vi "Open Handler.vi"(8 "error in (no error)":errorcluster, 10 "Configure Server":T1={"Outgoing Mail Server (SMTP)"="smtp.gmail.com", "Port"="587", "Sender's Email Address"="ltt24012025@gmail.com", "username"="ltt24012025@gmail.com", "password"="nftv\\swtbe\\suutg\\scqps", "Enable TLS"=TRUE}, 11 "Mail in":refnum<class "Mail.lvclass">) -> (0 "error out":errorcluster, 3 "Mail out":refnum<class "Mail.lvclass">)   [LabVIEW 2023, in "HardwareAbstractionLayer_LVOOP.lvlib" / "Mail.lvclass"]
uses:
  Mail.lvclass
  Mail.lvclass/Mail.ctl
  <vilib>/smtpClient/LabVIEWSMTPClient.lvlib
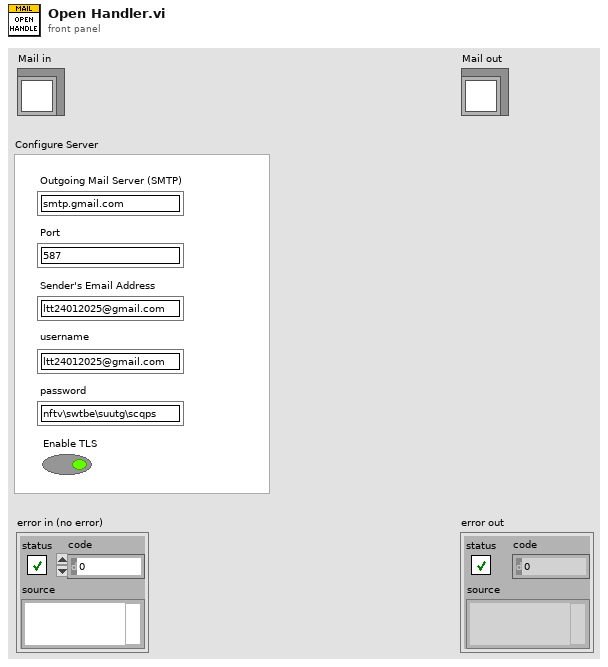
[diagram p1: front panel]
types:
  T1 = cluster{"Outgoing Mail Server (SMTP)":string, "Port":string, "Sender's Email Address":string, "username":string, "password":string, "Enable TLS":bool}
  T2 = typedef "LabVIEWSMTPClient.lvlib/SmtpClientHandle.ctl" = refnum<k1>
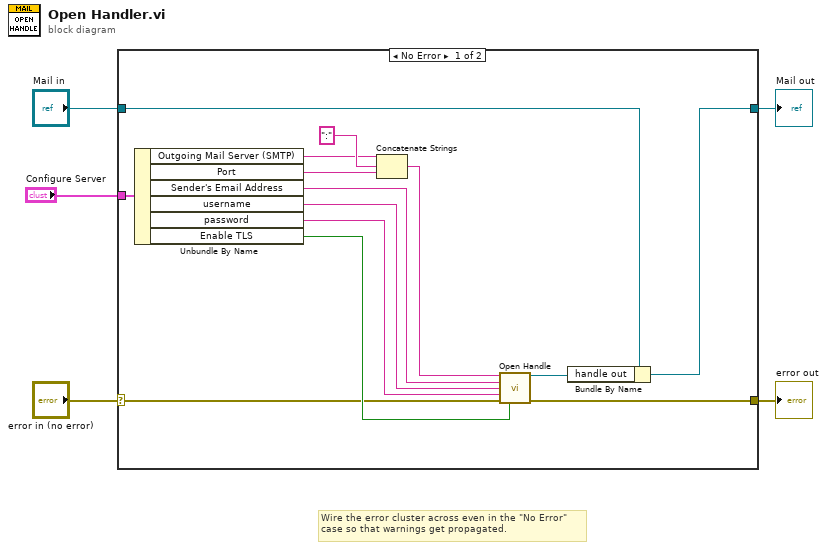
[diagram p0: block diagram]
diagram:
  # "Wire the error cluster across even in the \"No Error\"\ncase so that warnings get propagated."
  n1 = case shown="No Error" "error in (no error)" {
    selector: "error in (no error)" -> [w10 w21]
    tunnel: [w9 w21] -> w4
    tunnel: [w7 w20] -> w2
    tunnel: "Mail in" -> [w8 w20]
    tunnel: "Configure Server" -> [w17 _]
    frame No Error {
      n2 = Unbundle By Name(w17) -> ("Outgoing Mail Server (SMTP)"=w16:string, "Port"=w15:string, "Sender's Email Address"=w14:string, "username"=w13:string, "password"=w12:string, "Enable TLS"=w11:bool)
      n3 = Concatenate Strings(w16, ":" ("string"), w15) -> (w19:string)
      n4 = call <vilib>:"Open Handle.vi"("server address"=w19, "from"=w14, "username"=w13, "password"=w12, "error in (no error)"=w10, "use TLS (false)"=w11) -> ("handle out"=w6:T2, "error out"=w9:errorcluster)  [unwired: 8 in]
      n5 = Bundle By Name(cluster=w8, "handle out"=w6) -> (w7:refnum<class "Mail.lvclass">)
    }
    frame Error {
    }
  }
  "error out" <- w4
  "Mail out" <- w2
